vi "export Data 3D.vi"(4 "error in (no error)":errorcluster, 5 "Path":path, 6 "Data 2D Export Format Selection":T1, 7 "Data in":refnum<class "Data.lvclass">) -> (0 "error out":errorcluster, 3 "Data out":refnum<class "Data.lvclass">)   [LabVIEW 2018]
uses:
  SpectralRadar/LabVIEW/2012/user.lib/SpectralRadar.llb/Data.lvclass
  SpectralRadar/LabVIEW/2012/user.lib/SpectralRadar.llb/Data 3D Export Format Selection.ctl
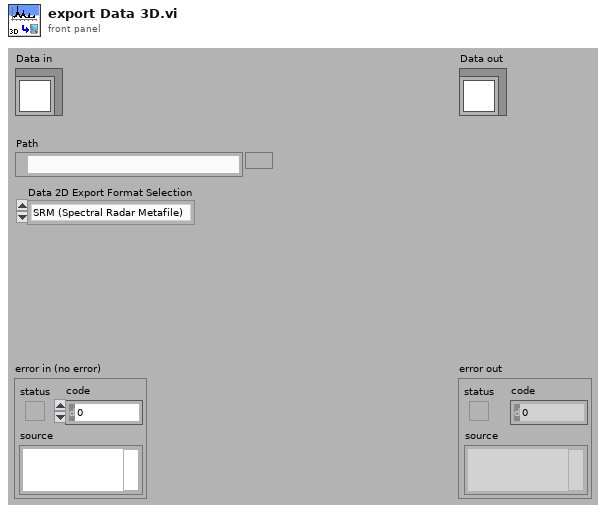
[diagram p1: front panel]
types:
  T1 = typedef "Data.lvclass/Data 3D Export Format Selection.ctl" = enum16{"SRM (Spectral Radar Metafile)", "RAW", "VFF", "VTK", "FITS"}
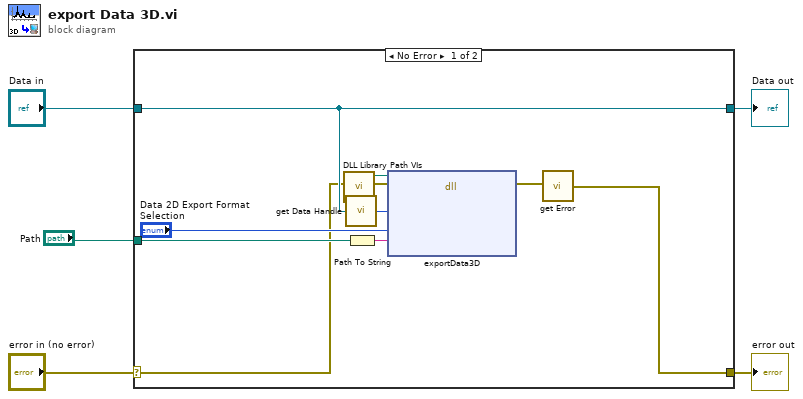
[diagram p0: block diagram]
diagram:
  n1 = case shown="No Error" "error in (no error)" {
    selector: "error in (no error)" -> [w7 w16]
    tunnel: [w8 w16] -> w4
    tunnel: [w13 w15] -> w2
    tunnel: "Data in" -> [w13 w15]
    tunnel: "Path" -> [w10 _]
    frame No Error {
      n2 = call "DLL Library Path VIs.vi"() -> ("SpectralRadarDLL"=w6:path)  [unwired: 8 in, 3 out]
      n3 = call "get Data Handle.vi"("Data"=w13) -> ("Handle"=w14:u64)
      n4 = Path To String(path=w10) -> (string=w12:string)
      n5 = dll-call lib="C:/Project/SerialSectOCT - FFT GPU/SerialSectOCT/Labview Software/DLL/SpectralRadar.dll" fn="exportData3D"(path in=w6, error in=w7, "Data Handle"=w14, "Volume Export Format"="Data 2D Export Format Selection", "File Name"=w12) -> (error out=w9:errorcluster)  [unwired: 5 in, 1 out]
      n6 = call "get Error.vi"("error in (no error)"=w9) -> ("error out"=w8:errorcluster)
    }
    frame Error {
    }
  }
  "error out" <- w4
  "Data out" <- w2
